vi "Criar nova lista de usuários.vi"(2 "Path":path) -> (0 "error out":errorcluster, 1 "file path":path)   [LabVIEW 2020]
uses:
  <vilib>/Utility/file.llb/Write Delimited Spreadsheet (string).vi
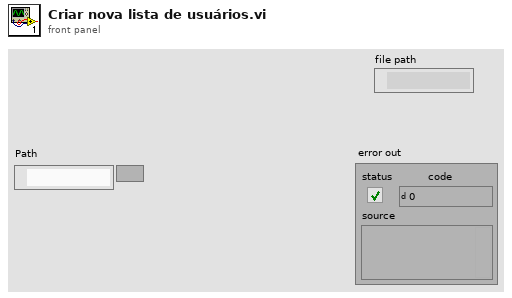
[diagram p1: front panel]
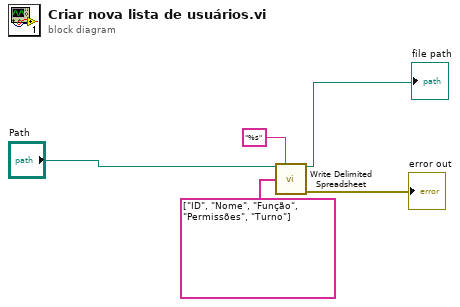
[diagram p0: block diagram]
diagram:
  n1 = call-poly <vilib>:"Write Delimited Spreadsheet.vi"("file path (dialog if empty)"="Path", "format (%s)"="%s" ("format (%.3f)"), "1D data"=string[] ["ID", "Nome", "Função", "Permissões", "Turno"]) -> ("new file path (Not A Path if cancelled)"=→"file path":path, "error out"=→"error out":errorcluster)  [unwired: 11 in]
